vi "Report File Write.vi"(8 "error in (no error)":errorcluster, 10 "Open if not? (T)":bool=TRUE, 11 "Report File in":refnum<class "Report File.lvclass">) -> (0 "error out":errorcluster, 3 "Report File out":refnum<class "Report File.lvclass">)   [LabVIEW 2018, in "Report File.lvclass"]
uses:
  Report File.lvclass
  Report File.lvclass/Report File.ctl
  e9848872-33c4-4b08-a39e-f4e86bb0405d.vi
  64b9eee6-4c70-4f46-853e-cbbbd9621403.vi
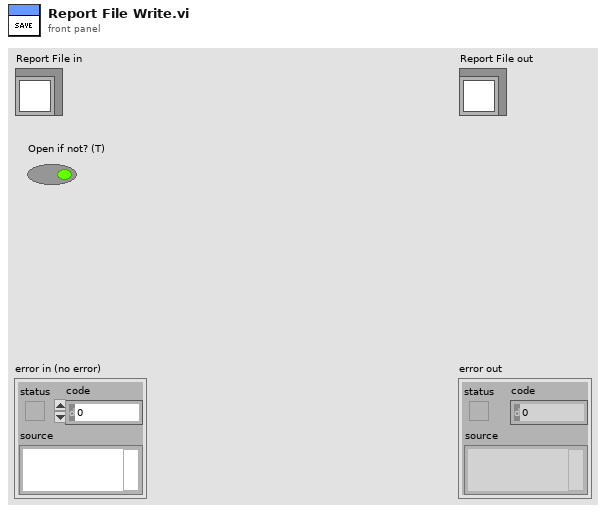
[diagram p1: front panel]
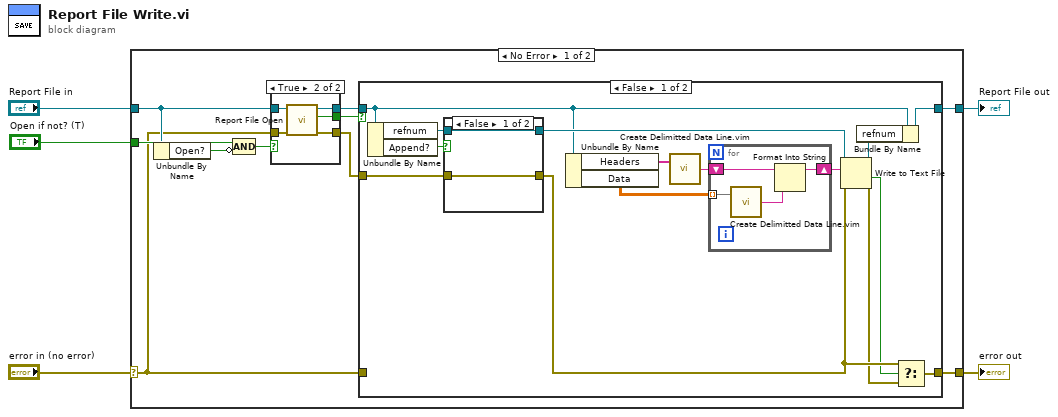
[diagram p0: block diagram]
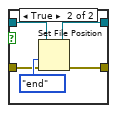
[diagram p2: hidden frame]
diagram:
  n1 = case shown="No Error" "error in (no error)" {
    selector: "error in (no error)" -> [w6 w52]
    tunnel: [w8 w52] -> w4
    tunnel: [w9 w51] -> w2
    tunnel: "Report File in" -> [w13 w51]
    tunnel: "Open if not? (T)" -> [w15 _]
    frame No Error {
      n2 = Unbundle By Name(w13) -> ("Open?"=w14:bool)
      n3 = Compound Arithmetic op=AND(w15, invert w14) -> (w12:bool)
      n4 = case shown="True" w12 {
        tunnel: w13 -> [w45 w50]
        tunnel: [w45 w49] -> w10
        tunnel: w6 -> [w44 w48]
        tunnel: [w44 w47] -> w11
        tunnel: [_ w46] -> w7
        frame False {
        }
        frame True {
          n5 = call-dynamic "Report File Open.vi"("error in (no error)"=w48, "Report File in"=w50) -> ("error out"=w47:errorcluster, "cancelled"=w46:bool, "Report File out"=w49:refnum<class "Report File.lvclass">)  [unwired: 7 in]
        }
      }
      n6 = case shown="False" w7 {
        tunnel: w11 -> [w28 _]
        tunnel: w10 -> [w22 w42]
        tunnel: [w20 w42] -> w9
        tunnel: [w17 w43] -> w8
        tunnel: w6 -> [_ w43]
        frame False {
          n7 = Unbundle By Name(w22) -> ("refnum"=w29:refnum<file>, "Append?"=w30:bool)
          n8 = case shown="False" w30 {
            tunnel: w29 -> [w36 w41]
            tunnel: w28 -> [w35 w39]
            tunnel: [w36 w38] -> w23
            tunnel: [w35 w37] -> w19
            frame False {
            }
            frame True {
              n9 = Set File Position(refnum=w41, from (0:start)=enum16{"start", "end", "current"}."end", error in=w39) -> (refnum out=w38:refnum<file>, error out=w37:errorcluster)  [unwired: 1 in]
            }
          }
          n10 = Unbundle By Name(w22) -> ("Headers"=w27:string[], "Data"=w26:dbl[][])
          n11 = call "Create Delimitted Data Line.vim"("Array"=w27) -> ("Delimitted Line"=w25:string)  [unwired: 1 in]
          n12 = for {
            tunnel: w26 -> [w34] mode=indexing
            shift-right: [w31] -> w24
            shift-left: w25 -> [w33]
            n13 = call "Create Delimitted Data Line.vim"("Array"=w34) -> ("Delimitted Line"=w32:string)  [unwired: 1 in]
            n14 = Format Into String(initial string=w33, w32) -> (resulting string=w31:string)  [unwired: 2 in, 1 out]
          }
          n15 = Write to Text File(file (use dialog)=w23, text=w24, error in=w19) -> (refnum out=w21:refnum<file>, cancelled=w16:bool, error out=w18:errorcluster)  [unwired: 1 in]
          n16 = Bundle By Name(cluster=w22, "refnum"=w21) -> (w20:refnum<class "Report File.lvclass">)
          n17 = Select(t=w19, s=w16, f=w18) -> (s? t:f=w17:errorcluster)
        }
        frame True {
        }
      }
    }
    frame Error {
    }
  }
  "error out" <- w4
  "Report File out" <- w2
